vi "KML-RenameSave.vi"(11 "path to vi or exe install\\data\\ dir":path) -> ()   [LabVIEW 8.6]
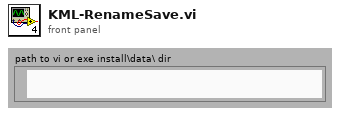
[diagram p1: front panel]
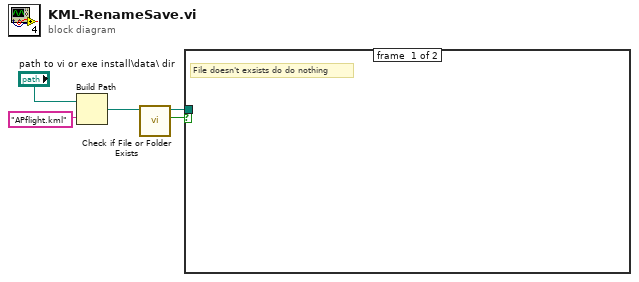
[diagram p0: block diagram]
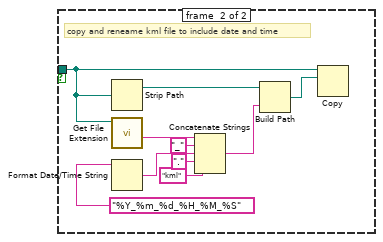
[diagram p2: hidden frame]
diagram:
  n1 = Build Path(base path="path to vi or exe install\\data\\ dir", name or relative path="APflight.kml") -> (appended path=w3:path)
  n2 = call <vilib>:"Check if File or Folder Exists.vi"("path"=w3) -> ("file or folder exists?"=w4:bool, "dup path"=w5:path)  [unwired: 8 in, 1 out]
  n3 = case shown="True" w4 {
    tunnel: w5 -> [_ w6]
    frame #0 {
      # "File doesn't exsists do do nothing"
    }
    frame #1 {
      # "copy and reneame kml file to include date and time"
      n4 = Strip Path(path=w6) -> (stripped path=w7:path)  [unwired: 1 out]
      n5 = call <vilib>:"Get File Extension.vi"("file"=w6) -> ("filename without extension"=w14:string)  [unwired: 7 in, 3 out]
      n6 = Format Date/Time String(time format string (%c)="%Y_%m_%d_%H_%M_%S") -> (date/time string=w12:string)  [unwired: 2 in]
      n7 = Concatenate Strings(w14, "_" ("string"), w12, "." ("string"), "kml" ("string")) -> (w8:string)
      n8 = Build Path(base path=w7, name or relative path=w8) -> (appended path=w9:path)
      n9 = Copy(10:w9, 11:w6) -> ()  [unwired: 3 in, 3 out]
    }
  }
